vi "Configure Sweep Coupling.vi"(4 "sweep time":dbl caption="sweep time (sec)", 5 "sweep time auto (Off)":bool, 6 "video bandwidth":dbl caption="video bandwidth (Hz)", 7 "video bandwidth auto (Off)":bool, 8 "error in (no error)":errorcluster {"code" format="%.0x"}, 9 "resolution bandwidth":dbl caption="resolution bandwidth (Hz)", 10 "resolution bandwidth auto (Off)":bool, 11 "instrument handle":refnum<k15>) -> (0 "error out":errorcluster {"code" format="%.0x"}, 3 "instrument handle out":refnum<k15>)   [LabVIEW 2009, in "Keysight XSAn.lvlib"]
doc: "This VI configures the coupling and sweeping properties of the IviSpecAn.\n\nSupported Models: M9290A, N8973B, N8974B, N8975B, N8976B, N9000A, N9000B, N9010A, N9010B, N9020A, N9020B, N9030A, N9030B, N9038A, N9040B, N9041B, SPN9003A, SPN9026A"
uses:
  <instrlib>/Keysight XSAn/Keysight XSAn.lvlib
  AgXSAn.dll
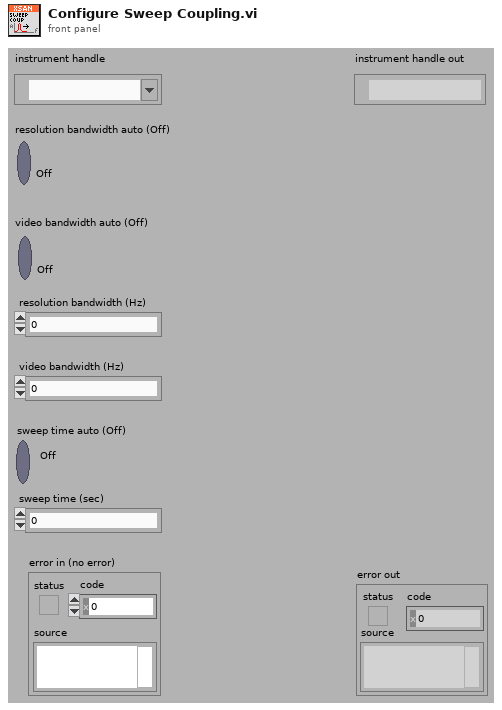
[diagram p1: front panel]
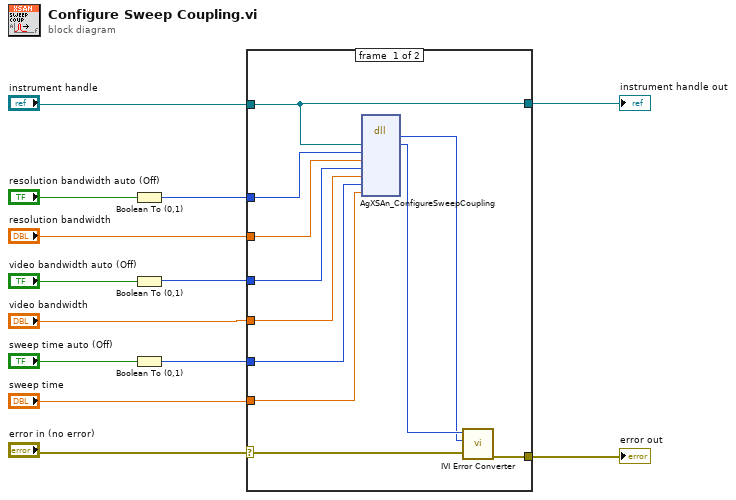
[diagram p0: block diagram]
diagram:
  n1 = Boolean To (0,1)(Boolean="resolution bandwidth auto (Off)") -> (0, 1=w1:i16)
  n2 = Boolean To (0,1)(Boolean="video bandwidth auto (Off)") -> (0, 1=w3:i16)
  n3 = Boolean To (0,1)(Boolean="sweep time auto (Off)") -> (0, 1=w5:i16)
  n4 = case shown="No Error" "error in (no error)" {
    selector: "error in (no error)" -> [w22 w26]
    tunnel: [w23 w26] -> w12
    tunnel: "instrument handle" -> [w21 w25]
    tunnel: [w21 w25] -> w10
    tunnel: "sweep time" -> [w19 _]
    tunnel: w5 -> [w18 _]
    tunnel: "video bandwidth" -> [w17 _]
    tunnel: w3 -> [w16 _]
    tunnel: "resolution bandwidth" -> [w15 _]
    tunnel: w1 -> [w14 _]
    frame #0 {
      n5 = dll-call lib="AgXSAn**.dll" fn="AgXSAn_ConfigureSweepCoupling" ("LabVIEW:IviSpecAn_ConfigureSweepCoupling")("instrument handle"=w21, "resolution bandwidth auto"=w14, "resolution bandwidth"=w15, "video bandwidth auto"=w16, "video bandwidth"=w17, "sweep time auto"=w18, "sweep time"=w19) -> ("Status"=w20:i32, "instrument handle"=w24:u32)  [unwired: 9 in, 2 out]
      n6 = call <instrlib>:"IVI Error Converter.vi"("error in (no error)"=w22, "IVI error code (0)"=w20, "instrument handle"=w24) -> ("error out"=w23:errorcluster)  [unwired: 7 in, 1 out]
    }
    frame #1 {
    }
  }
  "error out" <- w12
  "instrument handle out" <- w10
